vi "inverse_kin_objective_fn.vi"(3 "output control":T1, 4 "data":T2, 5 "X":dbl[](array[numeric])) -> (0 "error out":errorcluster, 1 "gradient":dbl[](array[numeric]), 2 "f(X)":dbl)   [LabVIEW 2025]
doc: "This template is the starting point for creating an objectivel function to be passed to the Unconstrained Optimization.vi."
uses:
  <vilib>/gmath/NumericalOptimization/objective function data.ctl
  <vilib>/Analysis/Matrix/Numeric/Subtract/Subtract - RM,RM.vi
  <vilib>/Analysis/Matrix/NI_Matrix.lvlib
  <vilib>/gmath/NI_Gmath.lvlib
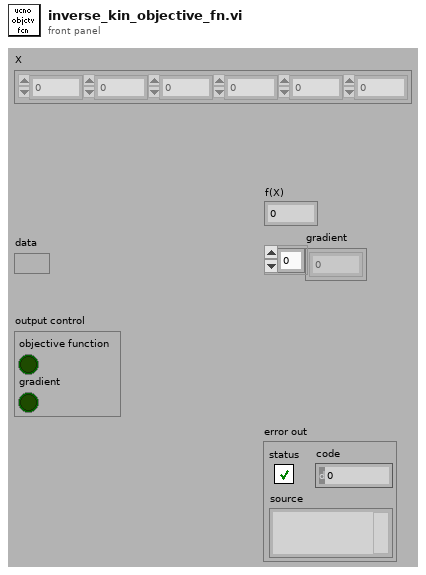
[diagram p1: front panel]
types:
  T1 = cluster{"objective function":bool, "gradient":bool}
  T2 = typedef "NI_Gmath.lvlib/objective function data.ctl" = variant
  T3 = typedef "NI_Matrix.lvlib/RealMatrix.ctl" = dbl[][]
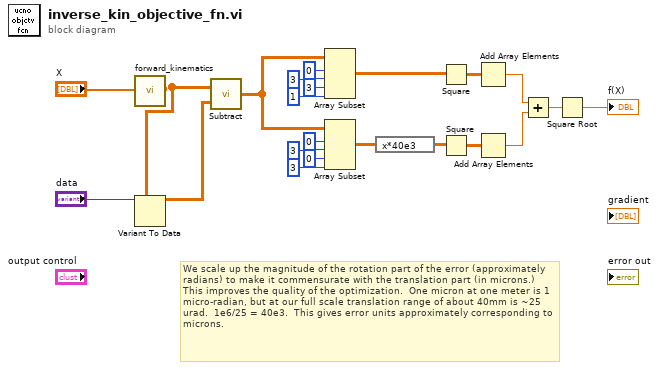
[diagram p0: block diagram]
diagram:
  # "We scale up the magnitude of the rotation part of the error (approximately radians) to make it commensurate with the translation part (in microns.)  This improves the quality of the optimization.  One micron at one meter is 1 micro-radian, but at our full scale translation range of about 40mm is ~25 urad.  1e6/25 = 40e3.  This gives error units approximately corresponding to microns."
  n1 = call "forward_kinematics.vi"("Axis positions"="X") -> ("Pose"=w15:T3)  [unwired: 10 in]
  n2 = Variant To Data(type=w15, Variant="data") -> (data=w14:T3)  [unwired: 1 in, 1 out]
  n3 = call-poly <vilib>:"Subtract.vi"("Real Matrix B"=w14, "Real Matrix A"=w15) -> ("A - B"=w9:T3)
  n4 = Array Subset(array=w9, index (row)=0 ("index"), length (row)=3 ("length"), index (col)=3 ("index"), length (col)=1 ("length")) -> (w5:T3)
  n5 = Array Subset(array=w9, index (row)=0 ("index"), length (row)=3 ("length"), index (col)=0 ("index"), length (col)=3 ("length")) -> (w8:T3)
  n6 = expression code="x*40e3"(w8) -> (w7:T3)
  n7 = Square(x=w5) -> (x^2=w6:T3)
  n8 = Square(x=w7) -> (x^2=w20:T3)
  n9 = Add Array Elements(numeric array=w6) -> (sum=w3:dbl)
  n10 = Add Array Elements(numeric array=w20) -> (sum=w4:dbl)
  n11 = Add(x=w3, y=w4) -> (x+y=w2:dbl)
  n12 = Square Root(x=w2) -> (sqrt(x)=→"f(X)":dbl)
